vi "read_params.vi"(8 "error in (no error)":errorcluster, 11 "NuSVR in":refnum<class "NuSVR.lvclass">) -> (0 "error out":errorcluster, 2 "params":T1={"nu"=0.5, "C"=1.0, "kernel"="rbf", "degree"=3.0, "gamma"={"gamma_type"="scale", "gamma_float"=0.001}, "coef0"=0.0, "shrinking"=TRUE, "tol"=0.001, "cache_size"=200.0, "verbose"=FALSE, "max_iter"=-1.0}, 3 "NuSVR out":refnum<class "NuSVR.lvclass">)   [LabVIEW 2020, in "NuSVR.lvclass"]
uses:
  NuSVR.lvclass
  Controls/nu_svr_params.ctl
  NuSVR.lvclass/NuSVR.ctl
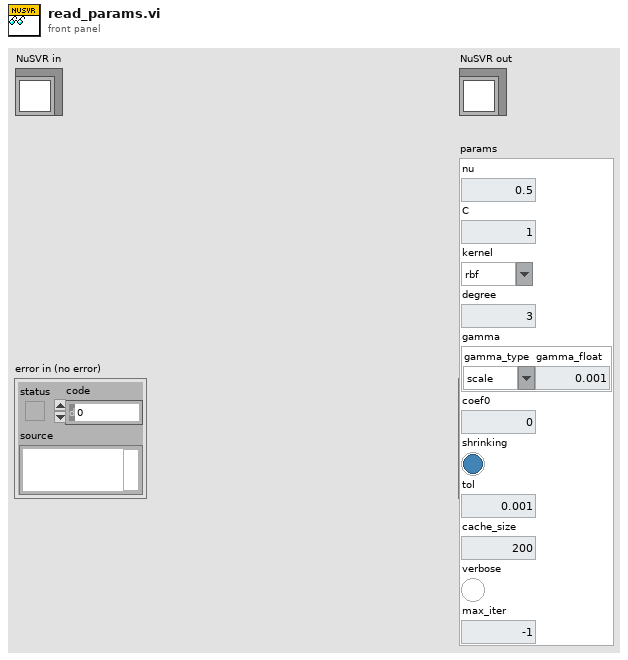
[diagram p1: front panel]
types:
  T1 = typedef "nu_svr_params.ctl" = cluster{"nu":dbl, "C":dbl, "kernel":string, "degree":dbl, "gamma":cluster{"gamma_type":string, "gamma_float":dbl}, "coef0":dbl, "shrinking":bool, "tol":dbl, "cache_size":dbl, "verbose":bool, "max_iter":dbl}
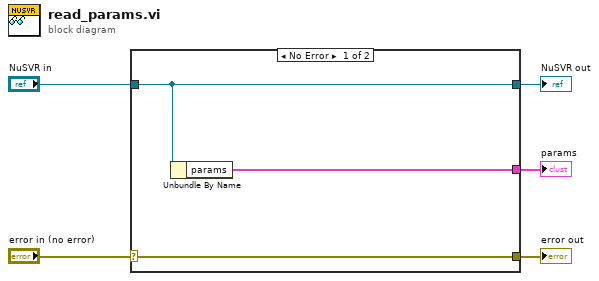
[diagram p0: block diagram]
diagram:
  n1 = case shown="No Error" "error in (no error)" {
    selector: "error in (no error)" -> [w8 w9]
    tunnel: [w8 w9] -> w4
    tunnel: [w7 w10] -> w2
    tunnel: "NuSVR in" -> [w7 w10]
    tunnel: [w6 _] -> w1
    frame No Error {
      n2 = Unbundle By Name(w7) -> ("params"=w6:T1)
    }
    frame Error {
    }
  }
  "error out" <- w4
  "NuSVR out" <- w2
  "params" <- w1
